vi "Log_Intrinsic_Data (SubVI).vi"(8 "error in (no error)":errorcluster, 11 "Intrinsic Data Cluster TD in":T1) -> (0 "error out":errorcluster)   [LabVIEW 2016]
uses:
  Intrinsic data TD.ctl
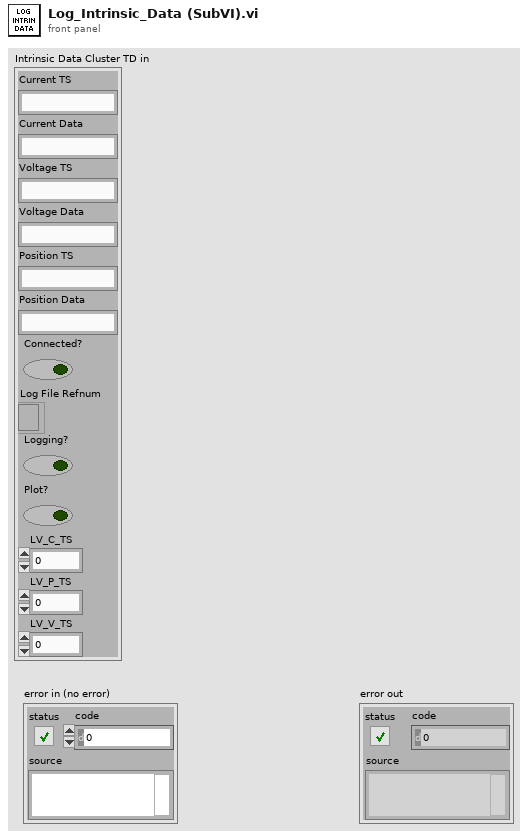
[diagram p1: front panel]
types:
  T1 = typedef "Intrinsic data TD.ctl" = cluster{"Current TS":string, "Current Data":string, "Voltage TS":string, "Voltage Data":string, "Position TS":string, "Position Data":string, "Connected?":bool, "Log File Refnum":refnum<file>, "Logging?":bool, "Plot?":bool, "LV_C_TS":dbl, "LV_P_TS":dbl, "LV_V_TS":dbl}
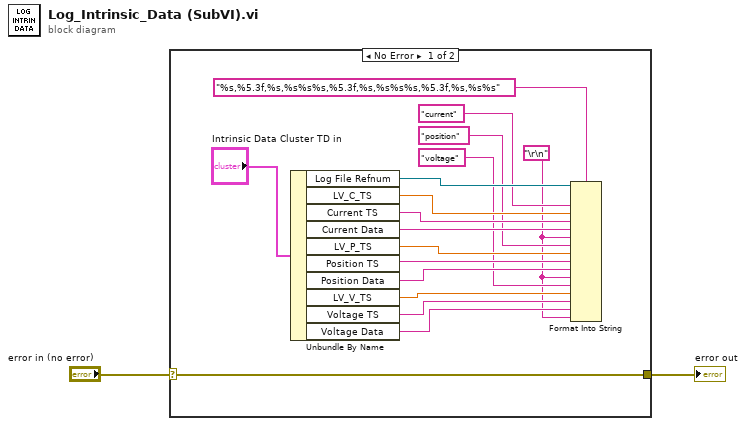
[diagram p0: block diagram]
diagram:
  n1 = case shown="No Error" "error in (no error)" {
    selector: "error in (no error)" -> [w17 w20]
    tunnel: [w17 w20] -> w1
    frame No Error {
      w3 = "\r\n"
      n2 = Unbundle By Name("Intrinsic Data Cluster TD in") -> ("Log File Refnum"=w19:refnum<file>, "LV_C_TS"=w14:dbl, "Current TS"=w13:string, "Current Data"=w12:string, "LV_P_TS"=w10:dbl, "Position TS"=w9:string, "Position Data"=w8:string, "LV_V_TS"=w6:dbl, "Voltage TS"=w5:string, "Voltage Data"=w4:string)
      n3 = Format Into String(format string="%s,%5.3f,%s,%s%s%s,%5.3f,%s,%s%s%s,%5.3f,%s,%s%s", initial string=w19, "current", w14, w13, w12, w3, "position", w10, w9, w8, w3, "voltage", w6, w5, w4, w3) -> ()  [unwired: 1 in, 2 out]
    }
    frame Error {
    }
  }
  "error out" <- w1
